vi "Read Library ref.vi"(8 "error in (no error)":errorcluster, 11 "HRF_Device in":refnum<class "HRF_Device.lvclass">) -> (0 "error out":errorcluster, 2 "Library ref":refnum<k24>, 3 "HRF_Device out":refnum<class "HRF_Device.lvclass">)   [LabVIEW 2020, in "HRF_Device.lvclass"]
uses:
  HRF_Device.lvclass
  D:/work/HackRF/Labview Driver/NetHackrf.dll
  NetHackrf.dll
  HRF_Device.lvclass/HRF_Device.ctl
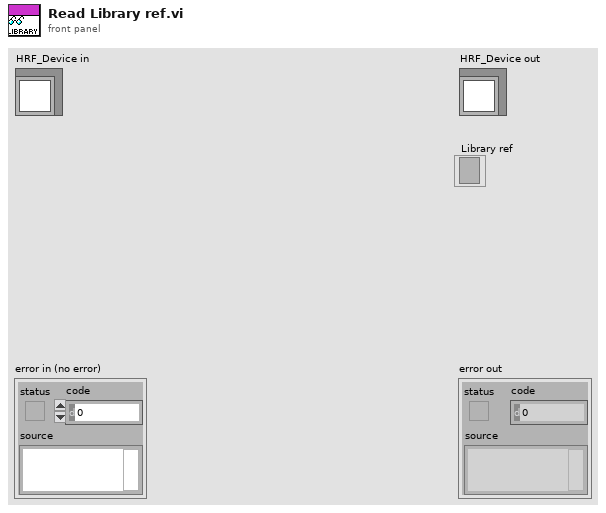
[diagram p1: front panel]
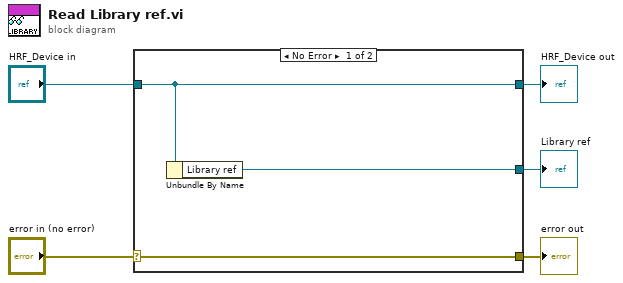
[diagram p0: block diagram]
diagram:
  n1 = case shown="No Error" "error in (no error)" {
    selector: "error in (no error)" -> [w8 w9]
    tunnel: [w8 w9] -> w4
    tunnel: [w7 w10] -> w2
    tunnel: "HRF_Device in" -> [w7 w10]
    tunnel: [w6 _] -> w1
    frame No Error {
      n2 = Unbundle By Name(w7) -> ("Library ref"=w6:refnum<k24>)
    }
    frame Error {
    }
  }
  "error out" <- w4
  "HRF_Device out" <- w2
  "Library ref" <- w1
